vi "Update Model Serial.vi"(8 "error in":errorcluster, 11 "Base Software in":refnum<class "Base Software.lvclass">) -> (0 "error out":errorcluster, 2 "Cancelled":bool, 3 "Base Software out":refnum<class "Base Software.lvclass">)   [LabVIEW 2019, in "Base Software.lvlib" / "Main.lvlib" / "Base Software.lvclass"]
uses:
  Project/Base Software.lvclass
  Project/Base Software.lvclass/Base Software.ctl
  Accessors/StateMachine/Write UUT_Info.vi
  Accessors/Indicators/Write Model.vi
  Accessors/Indicators/Write Serial.vi
  builds/Engine/Engine.lvlibp/Project/Engine.lvclass
  C:/Users/Public/Documents/Development/builds/Engine/Engine.lvlibp/Project/Engine.lvclass
panel:
  in  "Pedigree":enum16{"STAT", "BB", "PT", "EM", "FT"}(ring)
  out "String":string="Please enter a new model number and serial number:"
  in  "Cancel":bool
  in  "OK2":bool
  in  "Serial_Number":u16
  in  "Model":u16(ring) items=["STAT", "PSS", "PBC", "ABIS", "PCDA", "PDA", "MREU", "HCE"]
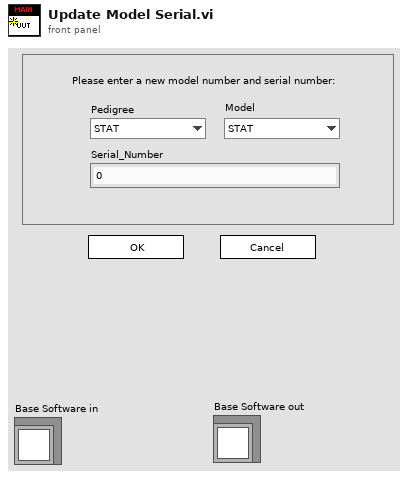
[diagram p1: front panel]
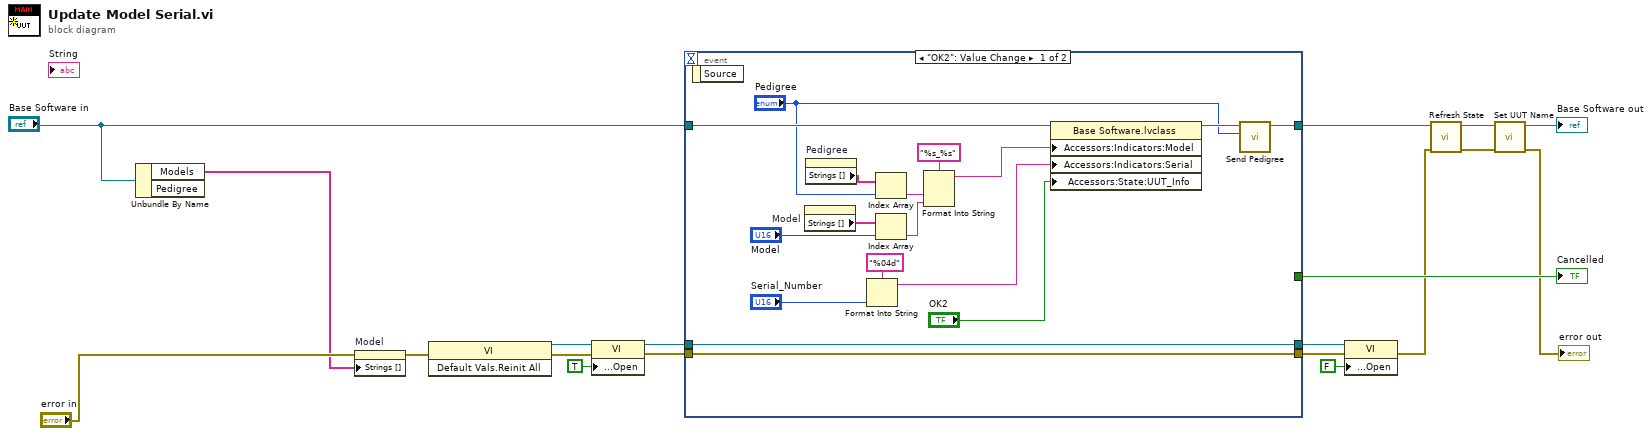
[diagram p0: block diagram]
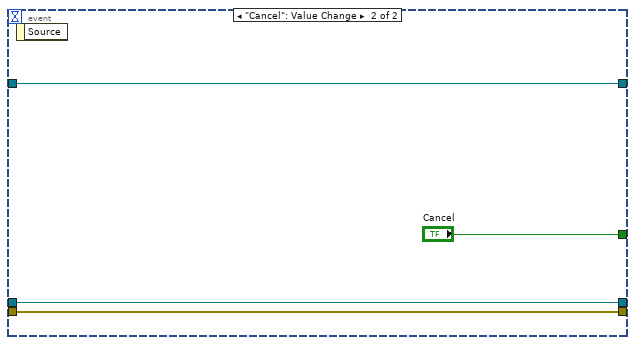
[diagram p2: hidden frame]
diagram:
  n1 = Unbundle By Name("Base Software in") -> ("Models"=w18:string[])  [unwired: 1 out]
  n2 = property on="Model" class="Ring (strict)"(error in="error in", "Strings []"=w18) -> (error out=w16:errorcluster)  [unwired: 1 in, 1 out]
  n3 = invoke class="VI" method="Default Vals.Reinit All"(error in=w16) -> (reference out=w17:refnum<vi>, error out=w15:errorcluster)  [unwired: 2 in, 1 out]
  n4 = property class="VI"(reference=w17, error in=w15, "Front Panel Window:Open"=TRUE) -> (reference out=w11:refnum<vi>, error out=w14:errorcluster)
  n5 = event shown="[0] \"OK2\": Value Change" {
    selector: _ -> [_ _]
    dyn-events: _ -> [_ _]
    timeout: _ -> [_ _]
    tunnel: "Base Software in" -> [w36 w40]
    tunnel: [w22 w40] -> w6
    tunnel: w14 -> [w26 w38]
    tunnel: [w26 w38] -> w12
    tunnel: w11 -> [w25 w39]
    tunnel: [w25 w39] -> w10
    tunnel: [_ "Cancel"] -> w7
    event "OK2": Value Change {
      n6 = event-data() -> ()  [unwired: 1 in, 1 out]
      n7 = property on="Model" class="Ring (strict)"() -> ("Strings []"=w33:string[])  [unwired: 2 in, 2 out]
      n8 = property on="Pedigree" class="Enum (strict)"() -> ("Strings []"=w20:string[])  [unwired: 2 in, 2 out]
      n9 = Format Into String(format string="%04d", "Serial_Number") -> (resulting string=w29:string)  [unwired: 2 in, 1 out]
      n10 = Index Array(array=w20, index="Pedigree") -> (element=w34:string)
      n11 = Index Array(array=w33, index="Model") -> (element=w32:string)
      n12 = Format Into String(format string="%s_%s", w34, w32) -> (resulting string=w31:string)  [unwired: 2 in, 1 out]
      n13 = property class="Base Software.lvclass"(reference=w36, "Accessors:Indicators:Model"=w31, "Accessors:Indicators:Serial"=w29, "Accessors:State:UUT_Info"="OK2") -> (reference out=w23:refnum<class "Base Software.lvclass">)  [unwired: 1 in, 1 out]
      n14 = call "Send Pedigree.vi"("Pedigree"="Pedigree", "Engine in"=w23) -> ("Engine out"=w22:refnum<class "Base Software.lvclass">)  [unwired: 8 in, 1 out]
    }
    event "Cancel": Value Change {
      n15 = event-data() -> ()  [unwired: 1 in, 1 out]
    }
  }
  "Cancelled" <- w7
  n16 = property class="VI"(reference=w10, error in=w12, "Front Panel Window:Open"=FALSE) -> (error out=w5:errorcluster)  [unwired: 1 out]
  n17 = call "Refresh State.vi"("error in"=w5, "Base Software in"=w6) -> ("error out"=w3:errorcluster, "Base Software out"=w4:refnum<class "Base Software.lvclass">)  [unwired: 8 in]
  n18 = call "Set UUT Name.vi"("error in"=w3, "Base Software in"=w4) -> ("error out"=→"error out":errorcluster, "Base Software out"=→"Base Software out":refnum<class "Base Software.lvclass">)  [unwired: 8 in]
